vi "FpgaInit.vi"(8 "error in (no error)":errorcluster, 11 "AODAcq in":refnum<class "AODAcq.lvclass">) -> (0 "error out":errorcluster, 3 "AODAcq out":refnum<class "AODAcq.lvclass">)   [LabVIEW 2012, in "AODAcq.lvclass"]
uses:
  AODAcq.lvclass
  <vilib>/userdefined/High Color/nirio_resource_hc.ctl
  <vilib>/LabVIEW Targets/FPGA/RIO/nirio_PxiTriggers.ctl
  <vilib>/FPGAPlugInAG/PXIe-7965R/niLvFpga_Open_PXIe-7965R.vi
  <vilib>/FPGAPlugInAG/PXIe-7965R/niLvFpga_Reset_PXIe-7965R.vi
  <vilib>/FPGAPlugInAG/PXIe-7965R/niLvFpga_Run_PXIe-7965R.vi
  <vilib>/LabVIEW Targets/FPGA/RIO/nirioReserveTrigger.vi
  <vilib>/LabVIEW Targets/FPGA/FlexRIO/CustomFPGAMethods/79XXR_Method_IOModuleStatusImpl.vi
  <vilib>/Utility/error.llb/Error Cluster From Error Code.vi
  <vilib>/rvi/errors/niLvFpgaAdjustHostInterfaceError.vi
  <vilib>/rvi/interface/nirviOpenFPGA/nirviOpenFPGA.xnode
  FPGA_Control/AODRef.ctl
  FPGA Bitfiles/AodScanner_FPGATarget_AODControl(FPGA)_HzWc4w5qqfg.lvbitx
  <vilib>/rvi/interface/nirviMethod/nirviMethod.xnode
  <vilib>/FPGA/interface/niFpgaViExecutionMode.ctl
  <vilib>/rvi/interface/nirviReadWriteControl/nirviReadWriteControl.xnode
  <vilib>/rvi/errors/niLvFpgaMergeErrorWithErrorCode.vi
  NiFpgaLv.dll
  <vilib>/FPGAPlugInAG/PXIe-7965R/niLvFpga_ConfigureFifo_PXIe-7965R.vi
  <vilib>/FPGAPlugInAG/PXIe-7965R/niLvFpga_StartFifo_PXIe-7965R.vi
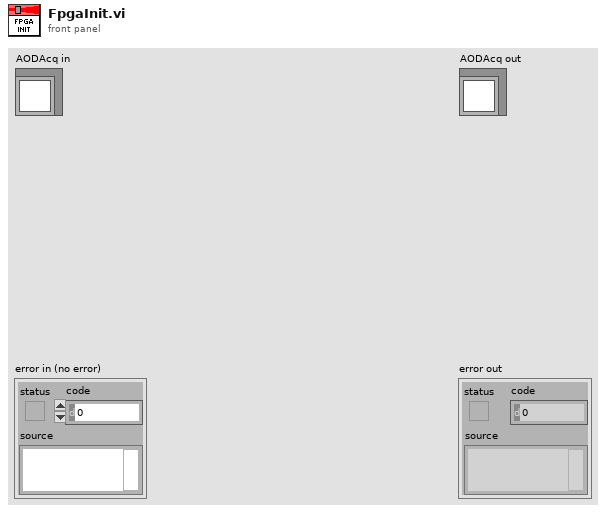
[diagram p1: front panel]
types:
  T1 = typedef "nirio_resource_hc.ctl" = tag
  T2 = typedef "AODRef.ctl" = refnum<k20>
  T3 = typedef "niFpgaViExecutionMode.ctl" = enum16{"FPGA Target", "Development Computer with Simulated I/O", "Development Computer with Real I/O", "Third-Party Simulator"}
  T4 = typedef "nirio_PxiTriggers.ctl" = u16
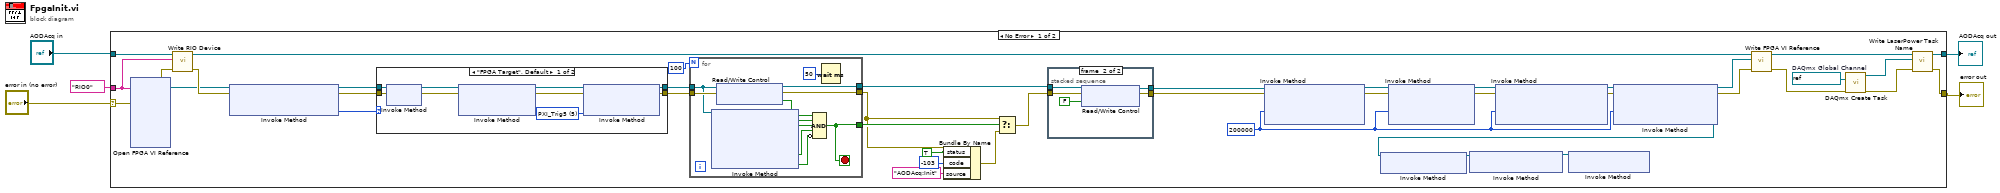
[diagram p0: block diagram]
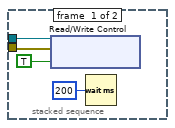
[diagram p2: hidden frame]
diagram:
  n1 = case shown="No Error" "error in (no error)" {
    selector: "error in (no error)" -> [w44 w79]
    tunnel: [w35 w79] -> w3
    tunnel: [w36 w78] -> w4
    tunnel: "AODAcq in" -> [w34 w78]
    tunnel: T1 "RIO0" ("RIO Device") -> [w32 _]
    frame No Error {
      w41 = refnum<k21> "AOD Gain"  # DAQmx Global Channel
      w13 = u32 200000 ("Depth")
      n2 = xnode "Open FPGA VI Reference"("error in"=w44, "resource name"=w32) -> ("FPGA VI Reference Out"=w6:T2, "error out"=w31:errorcluster)
      n3 = call-dynamic "Write RIO Device.vi"("error in (no error)"=w31, "RIO Device"=w32, "AODAcq in"=w34) -> ("error out"=w30:errorcluster, "AODAcq out"=w33:refnum<class "AODAcq.lvclass">)  [unwired: 7 in]
      n4 = xnode "Invoke Method"("FPGA VI Reference In"=w6, "error in"=w30) -> ("FPGA VI Reference Out"=w46:T2, "error out"=w43:errorcluster, "FPGA VI Execution Mode"=w45:T3)
      n5 = case shown="\"FPGA Target\", Default" w45 {
        tunnel: [w71 w77] -> w29
        tunnel: w46 -> [w75 w77]
        tunnel: w43 -> [w70 w76]
        tunnel: [w67 w76] -> w28
        frame "FPGA Target", Default {
          w73 = T4 5 items=["PXI_Trig0", "PXI_Trig1", "PXI_Trig2", "PXI_Trig3", "PXI_Trig4", "PXI_Trig5", "PXI_Trig6", "PXI_Trig7"] ("Trigger")
          n6 = xnode "Invoke Method"("FPGA VI Reference In"=w75, "error in"=w70) -> ("FPGA VI Reference Out"=w74:T2, "error out"=w69:errorcluster)
          n7 = xnode "Invoke Method"("FPGA VI Reference In"=w74, "error in"=w69) -> ("FPGA VI Reference Out"=w72:T2, "error out"=w68:errorcluster)  [unwired: 1 in]
          n8 = xnode "Invoke Method"("FPGA VI Reference In"=w72, "error in"=w68, "Trigger"=w73) -> ("FPGA VI Reference Out"=w71:T2, "error out"=w67:errorcluster)
        }
        frame "Development Computer with Simulated I/O" {
        }
      }
      n9 = for {
        N: 100 -> [_]
        tunnel: w29 -> [w56]
        tunnel: w28 -> [w57]
        tunnel: [w48] -> w27
        tunnel: [w50] -> w25
        tunnel: [w47] -> w20
        stop <- w48 stop-if-true
        n10 = xnode "Invoke Method"("FPGA VI Reference In"=w56) -> ("IO Module Present?"=w54:bool, "Power Enabled?"=w53:bool, "IO Enabled?"=w52:bool, "IO Module Mismatch?"=w51:bool)  [unwired: 1 in, 2 out]
        n11 = xnode "Read/Write Control"("FPGA VI Reference In"=w56, "error in"=w57) -> ("FPGA VI Reference Out"=w47:T2, "error out"=w50:errorcluster, "Status.Initialized"=w55:bool)
        n12 = Compound Arithmetic op=AND(w55, w54, w53, w52, invert w51) -> (w48:bool)
        n13 = Wait (ms)(milliseconds to wait=u32 50) -> ()  [unwired: 1 out]
      }
      n14 = Bundle By Name(cluster=w25, "status"=TRUE, "code"=-103, "source"="AODAcq:Init") -> (w24:errorcluster)
      n15 = Select(t=w25, s=w27, f=w24) -> (s? t:f=w19:errorcluster)
      n16 = stacked-sequence {
        tunnel: w20 -> [w61 w66]
        tunnel: w19 -> [w60 w65]
        tunnel: [_ w63] -> w8
        tunnel: [_ w62] -> w7
        frame #0 {
          n17 = xnode "Read/Write Control"("FPGA VI Reference In"=w61, "error in"=w60, "Control.Reset"=TRUE) -> ()  [unwired: 2 out]
          n18 = Wait (ms)(milliseconds to wait=u32 200) -> ()  [unwired: 1 out]
        }
        frame #1 {
          n19 = xnode "Read/Write Control"("FPGA VI Reference In"=w66, "error in"=w65, "Control.Reset"=FALSE) -> ("FPGA VI Reference Out"=w63:T2, "error out"=w62:errorcluster)
        }
      }
      n20 = xnode "Invoke Method"("FPGA VI Reference In"=w8, "error in"=w7, "Requested Depth"=w13) -> ("FPGA VI Reference Out"=w12:T2, "error out"=w42:errorcluster)  [unwired: 1 out]
      n21 = xnode "Invoke Method"("FPGA VI Reference In"=w12, "error in"=w42, "Requested Depth"=w13) -> ("FPGA VI Reference Out"=w18:T2, "error out"=w17:errorcluster)  [unwired: 1 out]
      n22 = xnode "Invoke Method"("FPGA VI Reference In"=w18, "error in"=w17, "Requested Depth"=w13) -> ("FPGA VI Reference Out"=w16:T2, "error out"=w15:errorcluster)  [unwired: 1 out]
      n23 = xnode "Invoke Method"("FPGA VI Reference In"=w16, "error in"=w15, "Requested Depth"=w13) -> ("FPGA VI Reference Out"=w11:T2, "error out"=w14:errorcluster)  [unwired: 1 out]
      n24 = xnode "Invoke Method"("FPGA VI Reference In"=w11) -> ("FPGA VI Reference Out"=w10:T2)  [unwired: 1 in, 1 out]
      n25 = xnode "Invoke Method"("FPGA VI Reference In"=w10) -> ("FPGA VI Reference Out"=w9:T2)  [unwired: 1 in, 1 out]
      n26 = xnode "Invoke Method"("FPGA VI Reference In"=w9) -> ()  [unwired: 1 in, 2 out]
      n27 = call-dynamic "Write FPGA VI Reference.vi"("error in (no error)"=w14, "AOD FPGA"=w11, "AODAcq in"=w33) -> ("error out"=w40:errorcluster, "AODAcq out"=w37:refnum<class "AODAcq.lvclass">)  [unwired: 7 in]
      n28 = call <vilib>:"DAQmx Create Task.vi"("global virtual channels"=w41, "error in"=w40) -> ("task out"=w38:refnum<k21>, "error out"=w39:errorcluster)  [unwired: 3 in, 9 out]
      n29 = call-dynamic "Write LaserPower Task Name.vi"("error in (no error)"=w39, "LaserPower Task Name"=w38, "AODAcq in"=w37) -> ("error out"=w35:errorcluster, "AODAcq out"=w36:refnum<class "AODAcq.lvclass">)  [unwired: 7 in]
    }
    frame Error {
    }
  }
  "error out" <- w3
  "AODAcq out" <- w4
